vi "Register Local Sub.vi"(8 "error in (no error)":errorcluster, 9 "Data Handler":refnum<class "SubscribedDataHandler.lvclass">, 10 "Group Name":string, 11 "VolatusAPI in":refnum<class "VolatusAPI.lvclass">) -> (0 "error out":errorcluster, 3 "VolatusAPI out":refnum<class "VolatusAPI.lvclass">)   [LabVIEW 2020, in "Volatus.lvlib" / "VolatusAPI.lvclass"]
uses:
  VolatusAPI.lvclass
  VolatusAPI.lvclass/VolatusAPI.ctl
  <vilib>/Utility/miscctls.llb/LVMapReplaceAction.ctl
  lv-vecto/Vecto/SubscribedDataHandler/SubscribedDataHandler.lvclass
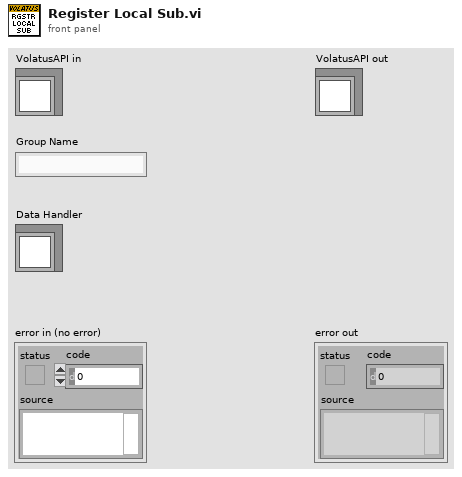
[diagram p1: front panel]
types:
  T1 = typedef "LVMapReplaceAction.ctl" = enum32{"Modify Entry only if found", "Add or Modify Entry", "Delete Entry"}
  T2 = map{string, refnum<class "SubscribedDataHandler.lvclass">[]}
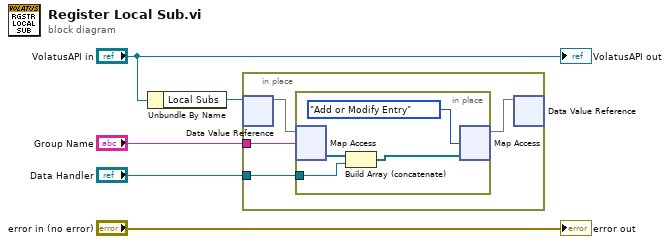
[diagram p0: block diagram]
diagram:
  n1 = Unbundle By Name("VolatusAPI in") -> ("Local Subs"=w4:refnum<data-value>)
  n2 = in-place {
    in-place-border: "Group Name" -> [w8]
    in-place-border: "Data Handler" -> [w7]
    n3 = in-place-dvr #1(w4) -> (w9:T2)  [unwired: 1 out]
    n4 = in-place {
      in-place-border: w7 -> [w12]
      n5 = in-place-map #2(w9, w8) -> (w13:refnum<class "SubscribedDataHandler.lvclass">[])  [unwired: 1 in, 1 out]
      n6 = Build Array (concatenate)(w13, w12) -> (w11:refnum<class "SubscribedDataHandler.lvclass">[])
      n7 = in-place-map #2(w11, LVMapReplaceAction."Add or Modify Entry" ("action")) -> (w6:T2)  [unwired: 2 out]
    }
    n8 = in-place-dvr #1(w6) -> ()  [unwired: 2 out]
  }
  "error out" <- "error in (no error)"
  "VolatusAPI out" <- "VolatusAPI in"
